vi "CalcRamUsage.vi"(7 "error in (no error)":errorcluster, 9 "nob":u32, 10 "nos":u32=6) -> (0 "error out":errorcluster, 3 "ramUsage":dbl=255.0)   [LabVIEW 2015, in "ESLSCDLL.lvlib"]
uses:
  ESLSCDLL.lvlib
  Globals.vi
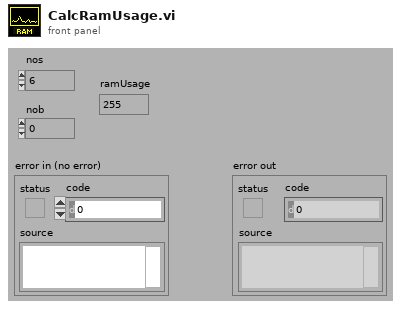
[diagram p1: front panel]
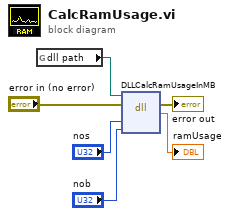
[diagram p0: block diagram]
diagram:
  n1 = global read "Globals.vi" "dll path"() -> (w1:path)
  n2 = dll-call lib="C:/ENTW/PCIE/LV64/board.vis/ESLSCDLL.dll" fn="DLLCalcRamUsageInMB" ("lwlscdll.dll:DLLReadLongS0")(path in=w1, error in="error in (no error)", "nos"="nos", "nob"="nob") -> (error out=→"error out":errorcluster, "Rückgabetyp"=→"ramUsage":dbl)  [unwired: 3 in, 1 out]
